vi "lasttime_rd.vi"(4 "error in":errorcluster, 6 "name or relative path":string="lasttime.txt", 7 "base path":path) -> (0 "error out":errorcluster, 2 "time stamp":timestamp, 3 "file path":path)   [LabVIEW 2010]
uses:
  <vilib>/Utility/miscctls.llb/LVDateTimeRec.ctl
panel:
  out "text":string
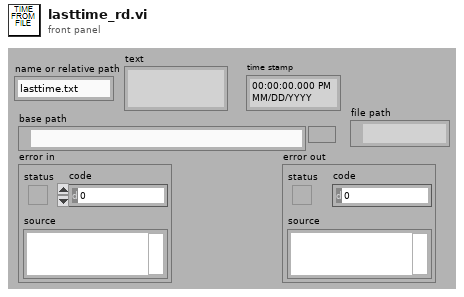
[diagram p1: front panel]
types:
  T1 = typedef "LVDateTimeRec.ctl" = cluster{"fractional second":dbl, "second":i32, "minute":i32, "hour":i32, "day of month":i32, "month":i32, "year":i32, "day of week":i32, "day of year":i32, "DST":i32}
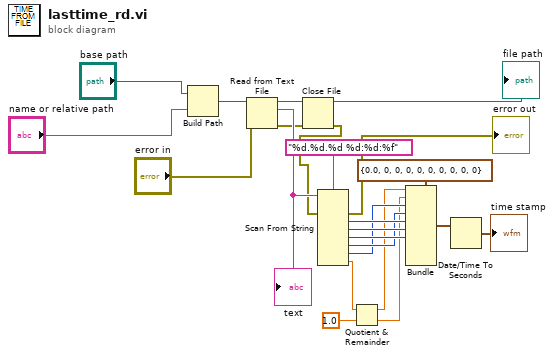
[diagram p0: block diagram]
diagram:
  n1 = Build Path(base path="base path", name or relative path="name or relative path") -> (appended path=w22:path)
  n2 = Read from Text File(file (use dialog)=w22, error in="error in") -> (refnum out=w11:refnum<file>, text=w21:string, error out=w12:errorcluster)  [unwired: 2 in, 1 out]
  "text" <- w21
  n3 = Close File(refnum=w11, error in=w12) -> (path=→"file path":path, error out=w6:errorcluster)
  n4 = Scan From String(format string="%d.%d.%d %d:%d:%f", input string=w21, error in=w6) -> (error out=→"error out":errorcluster, output 1=w16:i32, output 2=w18:i32, output 3=w17:i32, output 4=w15:i32, output 5=w14:i32, output 6=w4:dbl)  [unwired: 7 in, 2 out]
  n5 = Quotient & Remainder(x=w4, y=1.0) -> (x-y*floor(x/y)=w1:dbl, floor(x/y)=w2:dbl)
  n6 = Bundle(cluster=T1 {"fractional second"=0.0, "second"=0, "minute"=0, "hour"=0, "day of month"=0, "month"=0, "year"=0, "day of week"=0, "day of year"=0, "DST"=0} ("date time rec"), "fractional second"=w1, "second"=w2, "minute"=w14, "hour"=w15, "day of month"=w16, "month"=w18, "year"=w17) -> (w19:T1)  [unwired: 3 in]
  n7 = Date/Time To Seconds(2:w19) -> (0:→"time stamp":timestamp)  [unwired: 1 in]
